vi "UTILITY Release Semaphore.vi"(8 "error in (no error)":errorcluster, 9 "Debug":bool, 10 "Local?":bool, 11 "Refnum in":T1) -> (0 "error out":errorcluster)   [LabVIEW 2016]
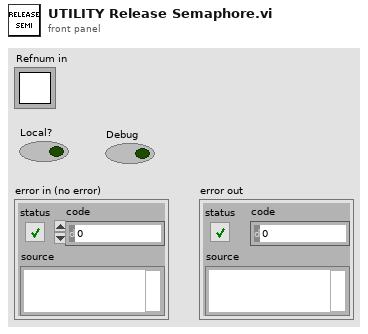
[diagram p1: front panel]
types:
  T1 = typedef "Semaphore RefNum" = refnum<k1>
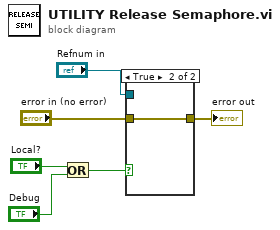
[diagram p0: block diagram]
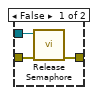
[diagram p2: hidden frame]
diagram:
  n1 = Or(x="Local?", y="Debug") -> (x .or. y?=w1:bool)
  n2 = case shown="True" w1 {
    tunnel: "error in (no error)" -> [w9 w10]
    tunnel: [w8 w10] -> w5
    tunnel: "Refnum in" -> [w7 _]
    frame False {
      n3 = call <vilib>:"Release Semaphore.vi"("error in (no error)"=w9, "semaphore"=w7) -> ("error out"=w8:errorcluster)  [unwired: 4 in, 1 out]
    }
    frame True {
    }
  }
  "error out" <- w5
